vi "Decompose LabVIEW Object - Private Data Indicator - Returns Private Data.vi"() -> ()   [LabVIEW 2017, in "Composition.Tests.lvlib"]
uses:
  Composition.Tests.lvlib
  Classes/Private Data Indicator/Private Data Indicator.lvclass
  Composition/Composition.lvlib
  <vilib>/addons/_JKI Toolkits/Caraya/classes/Assert/Assert.lvclass
  <vilib>/addons/_JKI Toolkits/Caraya/classes/Test/Test.lvclass
panel:
  out "error out":errorcluster
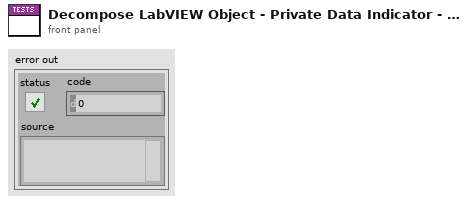
[diagram p1: front panel]
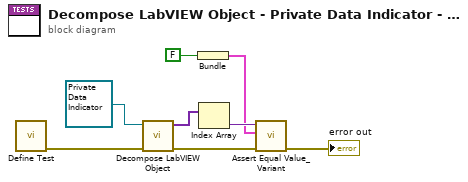
[diagram p0: block diagram]
diagram:
  n1 = call <vilib>:"Define Test.vi"() -> ("error out"=w4:errorcluster)  [unwired: 11 in]
  n2 = call "Decompose LabVIEW Object.vi"("error in (no error)"=w4, "LabVIEW Object"=refnum<class "Private Data Indicator.lvclass"> refnum ("Reflection.Tests.lvlib:Child.lvclass")) -> ("error out"=w7:errorcluster, "Private Data Clusters"=w5:variant[])  [unwired: 6 in, 2 out]
  n3 = Bundle(FALSE) -> (w1:cluster{bool})  [unwired: 1 in]
  n4 = Index Array(array=w5) -> (element=w3:variant)  [unwired: 1 in]
  n5 = call <vilib>:"Assert Equal Value_Variant.vi"("error in (no error)"=w7, "Y"=w1, "X"=w3) -> ("error out"=→"error out":errorcluster)  [unwired: 8 in]
